vi "AB_RW_Project_EXE_Info.vi"(7 "action":T1, 8 "error in (no error)":errorcluster, 10 "Exe_info in":T2, 11 "Object In":T5) -> (0 "error out":errorcluster, 2 "Exe info out":T2, 3 "Object Out":T5)   [LabVIEW 2020]
uses:
  <resource>/Framework/Providers/API/ItemRef.ctl
  <vilib>/AppBuilder/RW_Project/AB_RW_Project_EXE_Data.ctl
  <vilib>/AppBuilder/RW_Project/AB_RW_Project_EXE_SharedVar_Deploy.ctl
  <vilib>/AppBuilder/RW_Project/AB_RW_Project_EXE_SharedVar_LibInfo.ctl
  <vilib>/AppBuilder/RW_Project/AB_RW_Project_PropBag_Action.ctl
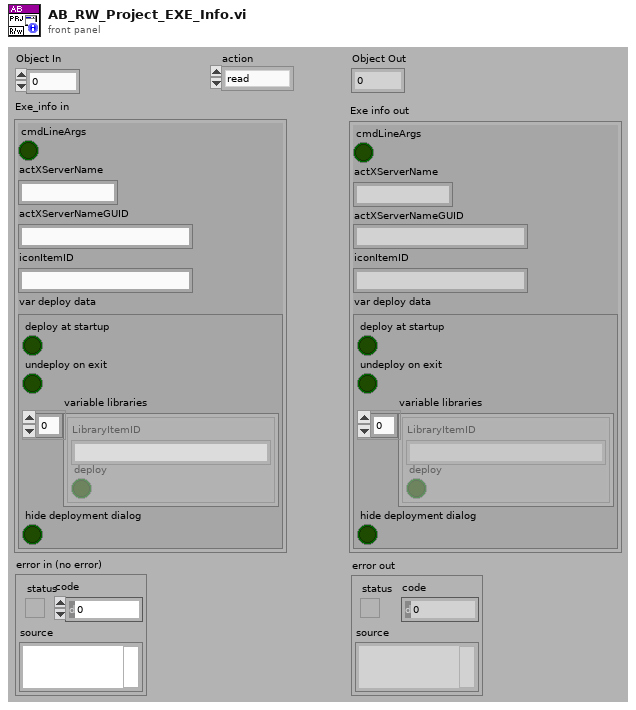
[diagram p1: front panel]
types:
  T1 = typedef "AB_RW_Project_PropBag_Action.ctl" = enum16{"read", "write", "clear", "readPrevious", "writePrevious", "clearPrevious"}
  T2 = typedef "AB_RW_Project_EXE_Data.ctl" = cluster{"cmdLineArgs":bool, "actXServerName":string, "actXServerNameGUID":string, "iconItemID":string, "var deploy data":T3}
  T3 = typedef "AB_RW_Project_EXE_SharedVar_Deploy.ctl" = cluster{"deploy at startup":bool, "undeploy on exit":bool, "variable libraries":T4[], "hide deployment dialog":bool}
  T4 = typedef "AB_RW_Project_EXE_SharedVar_LibInfo.ctl" = cluster{"LibraryItemID":string, "deploy":bool}
  T5 = typedef "ItemRef.ctl" = u64
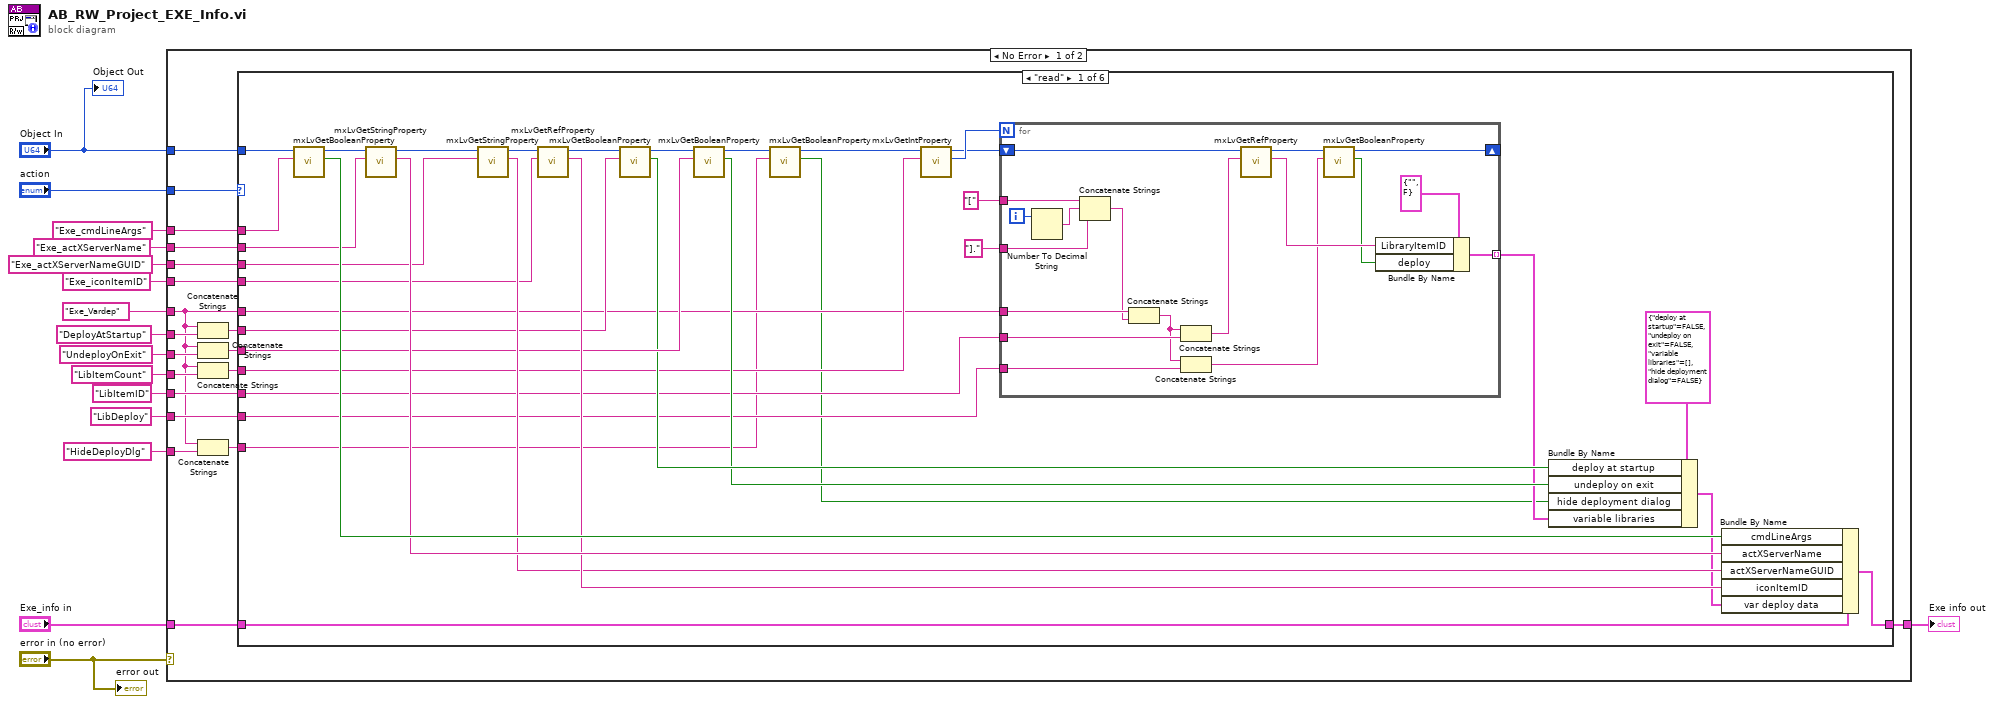
[diagram p0: block diagram]
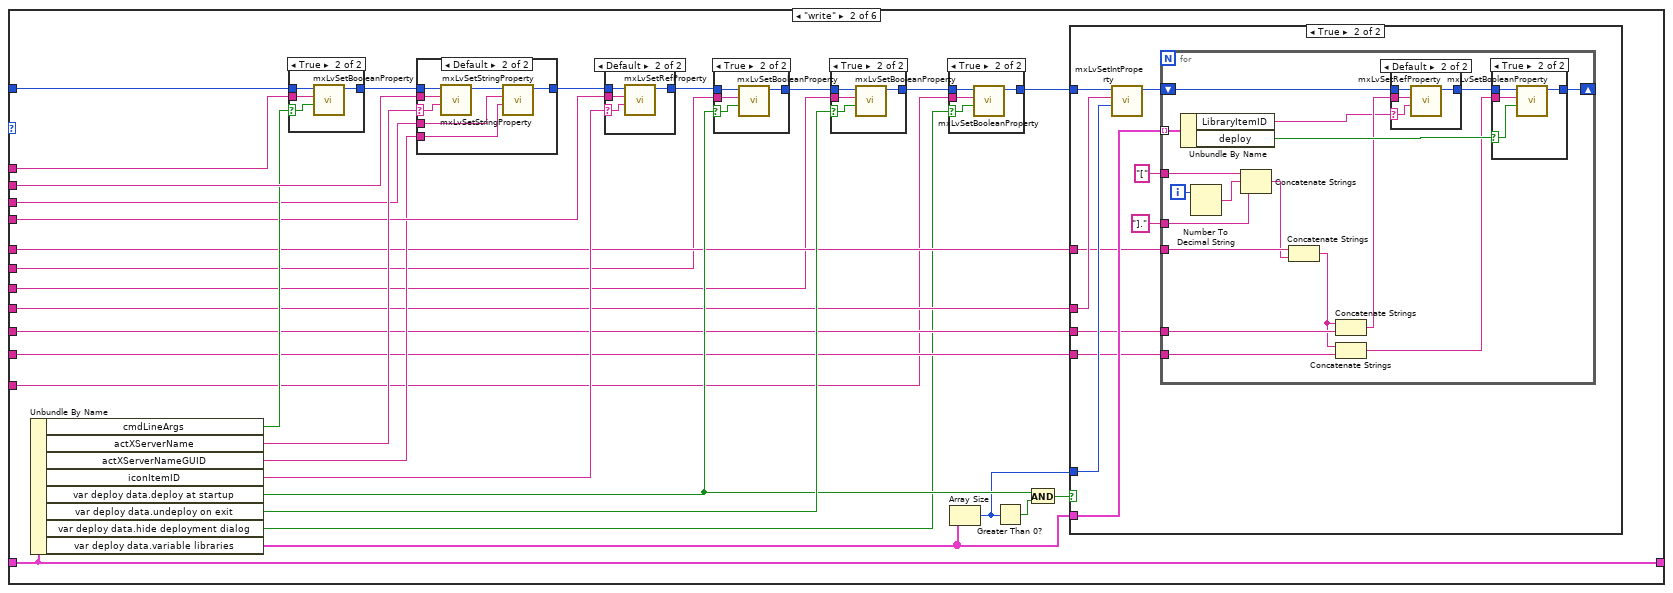
[diagram p2: hidden frame]
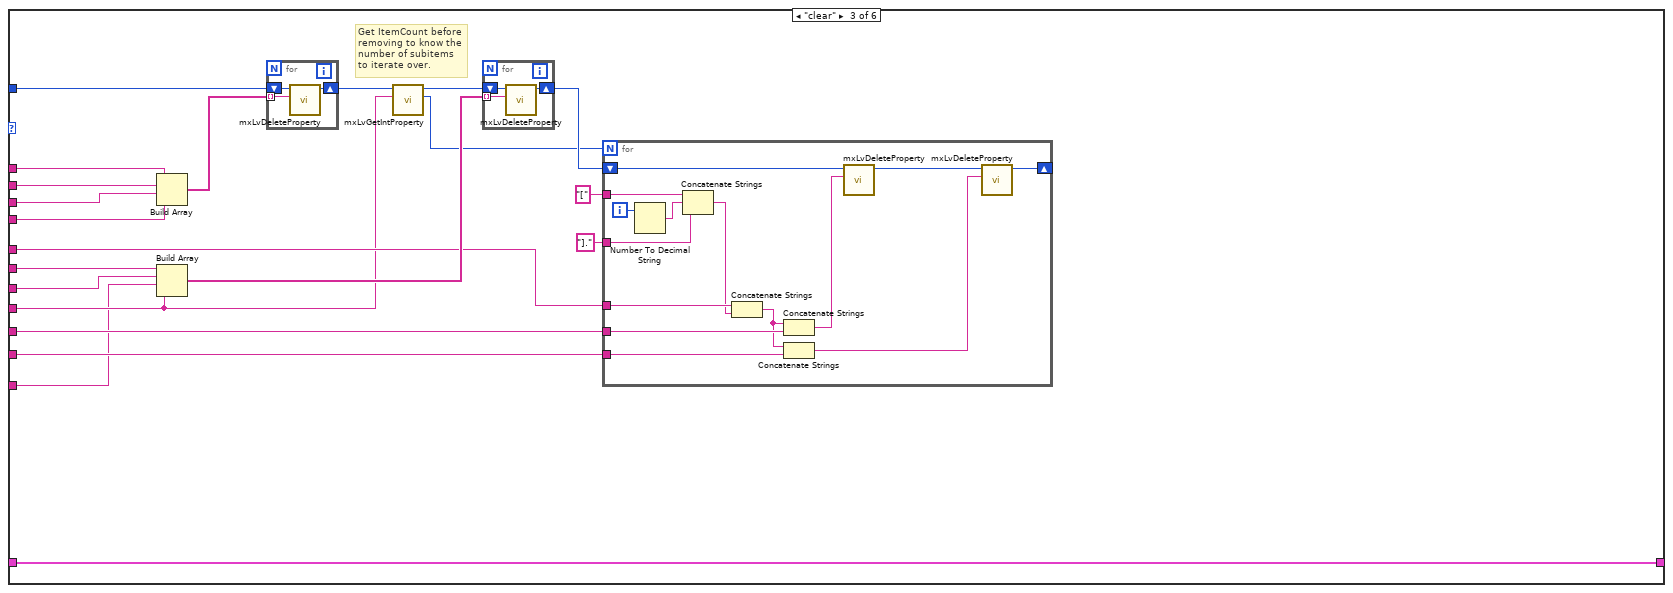
[diagram p12: hidden frame]
diagram:
  n1 = case shown="No Error" "error in (no error)" {
    tunnel: "Object In" -> [w33 _]
    tunnel: [w35 _] -> w14
    tunnel: "Exe_cmdLineArgs" -> [w34 _]
    tunnel: "Exe_actXServerName" -> [w32 _]
    tunnel: "Exe_actXServerNameGUID" -> [w31 _]
    tunnel: "Exe_info in" -> [w30 _]
    tunnel: "action" -> [w29 _]
    tunnel: "Exe_iconItemID" -> [w28 _]
    tunnel: "Exe_Vardep" -> [w18 _]
    tunnel: "DeployAtStartup" -> [w24 _]
    tunnel: "UndeployOnExit" -> [w23 _]
    tunnel: "LibItemCount" -> [w22 _]
    tunnel: "LibItemID" -> [w27 _]
    tunnel: "LibDeploy" -> [w26 _]
    tunnel: "HideDeployDlg" -> [w19 _]
    frame No Error {
      n2 = Concatenate Strings(w18, w24) -> (w21:string)
      n3 = Concatenate Strings(w18, w23) -> (w25:string)
      n4 = Concatenate Strings(w18, w22) -> (w20:string)
      n5 = Concatenate Strings(w18, w19) -> (w17:string)
      n6 = case shown="\"read\"" w29 {
        tunnel: [w66 w114 w209 w230 w231 w232] -> w35
        tunnel: w34 -> [w65 w113 w206 _ _ _]
        tunnel: w33 -> [w64 w118 w208 _ _ _]
        tunnel: w32 -> [w63 w115 w207 _ _ _]
        tunnel: w31 -> [w59 w107 w205 _ _ _]
        tunnel: w30 -> [w62 w114 w209 w230 w231 w232]
        tunnel: w28 -> [w57 w109 w203 _ _ _]
        tunnel: w18 -> [w43 w97 w193 _ _ _]
        tunnel: w21 -> [w54 w96 w200 _ _ _]
        tunnel: w25 -> [w52 w95 w199 _ _ _]
        tunnel: w20 -> [w49 w94 w190 _ _ _]
        tunnel: w27 -> [w42 w99 w192 _ _ _]
        tunnel: w26 -> [w41 w98 w191 _ _ _]
        tunnel: w17 -> [w37 w89 w189 _ _ _]
        frame "read" {
          n7 = call <resource>:"mxLvGetBooleanProperty.vi"("Tag"=w65, "Item"=w64) -> ("Value"=w69:bool, "Item"=w70:T5)  [unwired: 1 in, 7 out]
          n8 = call <resource>:"mxLvGetStringProperty.vi"("Tag"=w63, "Item"=w70) -> ("Value"=w68:string, "Item"=w61:T5)  [unwired: 1 in, 7 out]
          n9 = call <resource>:"mxLvGetStringProperty.vi"("Tag"=w59, "Item"=w61) -> ("Value"=w58:string, "Item"=w60:T5)  [unwired: 1 in, 7 out]
          n10 = call <resource>:"mxLvGetRefProperty.vi"("Tag"=w57, "Item"=w60) -> ("Value"=w67:string, "Item"=w46:T5)  [unwired: 1 in, 7 out]
          n11 = call <resource>:"mxLvGetBooleanProperty.vi"("Tag"=w54, "Item"=w46) -> ("Value"=w51:bool, "Item"=w53:T5)  [unwired: 1 in, 7 out]
          n12 = call <resource>:"mxLvGetBooleanProperty.vi"("Tag"=w52, "Item"=w53) -> ("Value"=w50:bool, "Item"=w39:T5)  [unwired: 1 in, 7 out]
          n13 = call <resource>:"mxLvGetBooleanProperty.vi"("Tag"=w37, "Item"=w39) -> ("Value"=w36:bool, "Item"=w38:T5)  [unwired: 1 in, 7 out]
          n14 = call <resource>:"mxLvGetIntProperty.vi"("Tag"=w49, "Item"=w38) -> ("Value"=w48:i32, "Item"=w47:T5)  [unwired: 1 in, 7 out]
          n15 = for {
            N: w48 -> [_]
            shift-right: [w88] -> _
            shift-left: w47 -> [w87]
            tunnel: "[" -> [w84]
            tunnel: "]." -> [w83]
            tunnel: w43 -> [w82]
            tunnel: w42 -> [w80]
            tunnel: w41 -> [w79]
            tunnel: [w76] -> w40 mode=indexing
            i -> [w85]
            n16 = Number To Decimal String(number=w85) -> (decimal integer string=w86:string)  [unwired: 1 out]
            n17 = Concatenate Strings(w84, w86, w83) -> (w81:string)
            n18 = Concatenate Strings(w82, w81) -> (w73:string)
            n19 = Concatenate Strings(w73, w80) -> (w78:string)
            n20 = Concatenate Strings(w73, w79) -> (w74:string)
            n21 = call <resource>:"mxLvGetRefProperty.vi"("Tag"=w78, "Item"=w87) -> ("Value"=w77:string, "Item"=w71:T5)  [unwired: 1 in, 7 out]
            n22 = call <resource>:"mxLvGetBooleanProperty.vi"("Tag"=w74, "Item"=w71) -> ("Value"=w75:bool, "Item"=w88:T5)  [unwired: 1 in, 7 out]
            n23 = Bundle By Name(cluster=T4 {"LibraryItemID"="", "deploy"=FALSE} ("variable libraries"), "LibraryItemID"=w77, "deploy"=w75) -> (w76:T4)
          }
          n24 = Bundle By Name(cluster=T3 {"deploy at startup"=FALSE, "undeploy on exit"=FALSE, "variable libraries"=[], "hide deployment dialog"=FALSE} ("var deploy data"), "deploy at startup"=w51, "undeploy on exit"=w50, "hide deployment dialog"=w36, "variable libraries"=w40) -> (w55:T3)
          n25 = Bundle By Name(cluster=w62, "cmdLineArgs"=w69, "actXServerName"=w68, "actXServerNameGUID"=w58, "iconItemID"=w67, "var deploy data"=w55) -> (w66:T2)
        }
        frame "write" {
          n26 = Unbundle By Name(w114) -> ("cmdLineArgs"=w112:bool, "actXServerName"=w111:string, "actXServerNameGUID"=w108:string, "iconItemID"=w110:string, "var deploy data.deploy at startup"=w103:bool, "var deploy data.undeploy on exit"=w104:bool, "var deploy data.hide deployment dialog"=w90:bool, "var deploy data.variable libraries"=w93:T4[])
          n27 = case shown="True" w112 {
            selector: w112 -> [_ w185]
            tunnel: w118 -> [w184 w188]
            tunnel: [w184 w187] -> w117
            tunnel: w113 -> [_ w186]
            frame False {
            }
            frame True {
              n28 = call <resource>:"mxLvSetBooleanProperty.vi"("Value (F)"=w185, "Tag"=w186, "Item"=w188) -> ("Item"=w187:T5)  [unwired: 2 in, 6 out]
            }
          }
          n29 = case shown="Default" w111 {
            selector: w111 -> [_ w181]
            tunnel: w117 -> [w176 w183]
            tunnel: [w176 w179] -> w116
            tunnel: w115 -> [_ w182]
            tunnel: w108 -> [_ w178]
            tunnel: w107 -> [_ w177]
            frame "" {
            }
            frame Default {
              n30 = call <resource>:"mxLvSetStringProperty.vi"("Value (\"\")"=w181, "Tag"=w182, "Item"=w183) -> ("Item"=w180:T5)  [unwired: 2 in, 6 out]
              n31 = call <resource>:"mxLvSetStringProperty.vi"("Value (\"\")"=w178, "Tag"=w177, "Item"=w180) -> ("Item"=w179:T5)  [unwired: 2 in, 6 out]
            }
          }
          n32 = case shown="Default" w110 {
            selector: w110 -> [_ w173]
            tunnel: w116 -> [w171 w175]
            tunnel: w109 -> [_ w174]
            tunnel: [w171 w172] -> w106
            frame "" {
            }
            frame Default {
              n33 = call <resource>:"mxLvSetRefProperty.vi"("Value (\"\")"=w173, "Tag"=w174, "Item"=w175) -> ("Item"=w172:T5)  [unwired: 2 in, 6 out]
            }
          }
          n34 = case shown="True" w103 {
            selector: w103 -> [_ w167]
            tunnel: w106 -> [w166 w170]
            tunnel: [w166 w169] -> w105
            tunnel: w96 -> [_ w168]
            frame False {
            }
            frame True {
              n35 = call <resource>:"mxLvSetBooleanProperty.vi"("Value (F)"=w167, "Tag"=w168, "Item"=w170) -> ("Item"=w169:T5)  [unwired: 2 in, 6 out]
            }
          }
          n36 = case shown="True" w104 {
            selector: w104 -> [_ w162]
            tunnel: w105 -> [w161 w165]
            tunnel: [w161 w164] -> w92
            tunnel: w95 -> [_ w163]
            frame False {
            }
            frame True {
              n37 = call <resource>:"mxLvSetBooleanProperty.vi"("Value (F)"=w162, "Tag"=w163, "Item"=w165) -> ("Item"=w164:T5)  [unwired: 2 in, 6 out]
            }
          }
          n38 = case shown="True" w90 {
            selector: w90 -> [_ w120]
            tunnel: w92 -> [w119 w123]
            tunnel: [w119 w122] -> w91
            tunnel: w89 -> [_ w121]
            frame False {
            }
            frame True {
              n39 = call <resource>:"mxLvSetBooleanProperty.vi"("Value (F)"=w120, "Tag"=w121, "Item"=w123) -> ("Item"=w122:T5)  [unwired: 2 in, 6 out]
            }
          }
          n40 = Array Size(array=w93) -> (size(s)=w100:i32)
          n41 = Greater Than 0?(x=w100) -> (x > 0?=w101:bool)
          n42 = And(x=w103, y=w101) -> (x .and. y?=w102:bool)
          n43 = case shown="True" w102 {
            tunnel: w91 -> [_ w133]
            tunnel: w93 -> [_ w129]
            tunnel: w94 -> [_ w132]
            tunnel: w100 -> [_ w131]
            tunnel: w99 -> [_ w125]
            tunnel: w98 -> [_ w124]
            tunnel: w97 -> [_ w128]
            frame False {
            }
            frame True {
              n44 = call <resource>:"mxLvSetIntProperty.vi"("Value (0)"=w131, "Tag"=w132, "Item"=w133) -> ("Item"=w130:T5)  [unwired: 2 in, 6 out]
              n45 = for {
                shift-right: [w148] -> _
                shift-left: w130 -> [w149]
                tunnel: w129 -> [w150] mode=indexing
                tunnel: w128 -> [w142]
                tunnel: "[" -> [w144]
                tunnel: "]." -> [w143]
                tunnel: w125 -> [w140]
                tunnel: w124 -> [w139]
                i -> [w145]
                n46 = Unbundle By Name(w150) -> ("LibraryItemID"=w135:string, "deploy"=w147:bool)
                n47 = Number To Decimal String(number=w145) -> (decimal integer string=w146:string)  [unwired: 1 out]
                n48 = Concatenate Strings(w144, w146, w143) -> (w141:string)
                n49 = Concatenate Strings(w142, w141) -> (w136:string)
                n50 = Concatenate Strings(w136, w140) -> (w138:string)
                n51 = Concatenate Strings(w136, w139) -> (w137:string)
                n52 = case shown="Default" w135 {
                  selector: w135 -> [_ w158]
                  tunnel: w149 -> [w156 w160]
                  tunnel: w138 -> [_ w159]
                  tunnel: [w156 w157] -> w134
                  frame "" {
                  }
                  frame Default {
                    n53 = call <resource>:"mxLvSetRefProperty.vi"("Value (\"\")"=w158, "Tag"=w159, "Item"=w160) -> ("Item"=w157:T5)  [unwired: 2 in, 6 out]
                  }
                }
                n54 = case shown="True" w147 {
                  selector: w147 -> [_ w152]
                  tunnel: w134 -> [w151 w155]
                  tunnel: [w151 w154] -> w148
                  tunnel: w137 -> [_ w153]
                  frame False {
                  }
                  frame True {
                    n55 = call <resource>:"mxLvSetBooleanProperty.vi"("Value (F)"=w152, "Tag"=w153, "Item"=w155) -> ("Item"=w154:T5)  [unwired: 2 in, 6 out]
                  }
                }
              }
            }
          }
        }
        frame "clear" {
          # "Get ItemCount before removing to know the number of subitems to iterate over."
          n56 = Build Array(w206, w207, w205, w203) -> (w204:string[])
          n57 = Build Array(w200, w199, w189, w190) -> (w198:string[])
          n58 = for {
            tunnel: w204 -> [w228] mode=indexing
            shift-right: [w227] -> w202
            shift-left: w208 -> [w229]
            n59 = call <resource>:"mxLvDeleteProperty.vi"("Tag"=w228, "Item"=w229) -> ("Item"=w227:T5)  [unwired: 1 in, 8 out]
          }
          n60 = call <resource>:"mxLvGetIntProperty.vi"("Tag"=w190, "Item"=w202) -> ("Value"=w194:i32, "Item"=w201:T5)  [unwired: 1 in, 7 out]
          n61 = for {
            tunnel: w198 -> [w225] mode=indexing
            shift-right: [w224] -> w195
            shift-left: w201 -> [w226]
            n62 = call <resource>:"mxLvDeleteProperty.vi"("Tag"=w225, "Item"=w226) -> ("Item"=w224:T5)  [unwired: 1 in, 8 out]
          }
          n63 = for {
            N: w194 -> [_]
            shift-right: [w223] -> _
            shift-left: w195 -> [w222]
            tunnel: "[" -> [w219]
            tunnel: "]." -> [w218]
            tunnel: w193 -> [w217]
            tunnel: w192 -> [w215]
            tunnel: w191 -> [w214]
            i -> [w220]
            n64 = Number To Decimal String(number=w220) -> (decimal integer string=w221:string)  [unwired: 1 out]
            n65 = Concatenate Strings(w219, w221, w218) -> (w216:string)
            n66 = Concatenate Strings(w217, w216) -> (w211:string)
            n67 = Concatenate Strings(w211, w215) -> (w213:string)
            n68 = Concatenate Strings(w211, w214) -> (w212:string)
            n69 = call <resource>:"mxLvDeleteProperty.vi"("Tag"=w213, "Item"=w222) -> ("Item"=w210:T5)  [unwired: 1 in, 8 out]
            n70 = call <resource>:"mxLvDeleteProperty.vi"("Tag"=w212, "Item"=w210) -> ("Item"=w223:T5)  [unwired: 1 in, 8 out]
          }
        }
        frame "writePrevious" {
        }
        frame "readPrevious" {
        }
        frame "clearPrevious" {
        }
      }
    }
    frame Error {
    }
  }
  "Exe info out" <- w14
  "Object Out" <- "Object In"
  "error out" <- "error in (no error)"
